vi "Time Zone Offset.vi"() -> ()   [LabVIEW 2010]
panel:
  in  "Offset":dbl
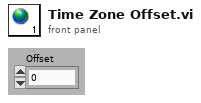
[diagram p1: front panel]
diagram:
